vi "TMP007 Read.vi"(7 "I2C Channel":u8, 8 "error in (no error)":errorcluster, 10 "I2C Slave Address":u8 format="%.0x", 11 "LINX Resource in":T2) -> (0 "error out":errorcluster, 1 "Conversion Time (S)":dbl format="%#_g s", 2 "Temp Readings":T1 {"Ambient Temp (°F)" format="%.2f °F"; "Ambient Temp (°C)" format="%.2f °C"; "Object Temp (°F)" format="%.2f °F"; "Object Temp (°C)" format="%.2f °C"}, 3 "LINX Resource":T2)   [LabVIEW 2014]
uses:
  <vilib>/MakerHub/LINX/Private/Type Defs/LINX Ref.ctl
  <vilib>/MakerHub/LINX/Private/Type Defs/Platform.ctl
  <vilib>/MakerHub/LINX/Private/Type Defs/Interface.ctl
  <vilib>/MakerHub/LINX/Private/Device/Type Defs/LINX Device Config.ctl
  <vilib>/MakerHub/LINX/Private/Device/Type Defs/TCP Config.ctl
  <vilib>/MakerHub/LINX/Private/Device/Type Defs/Channels.ctl
  <vilib>/MakerHub/LINX/Private/Local IO/LinxI2cWrite.vi
  <vilib>/MakerHub/LINX/Public/Utilities/Check Channel.vi
  <vilib>/myRIO/Instrument Drivers/Onboard IO/I2C/vis/Write.vi
  <vilib>/MakerHub/LINX/Private/Utilties/Generate Error.vi
  <vilib>/MakerHub/LINX/Private/Utilties/Channel FGVs/I2C Channels.vi
  <vilib>/Utility/error.llb/Error Cluster From Error Code.vi
  <vilib>/myRIO/Common/Instrument Driver Framework/myRIO v1.0/I2C/vis/myRIO v1.0 Write I2C.vi
  <vilib>/MakerHub/LINX/LMH-LINX.lvlib
  <vilib>/MakerHub/LINX/Private/Device/Device.lvlib
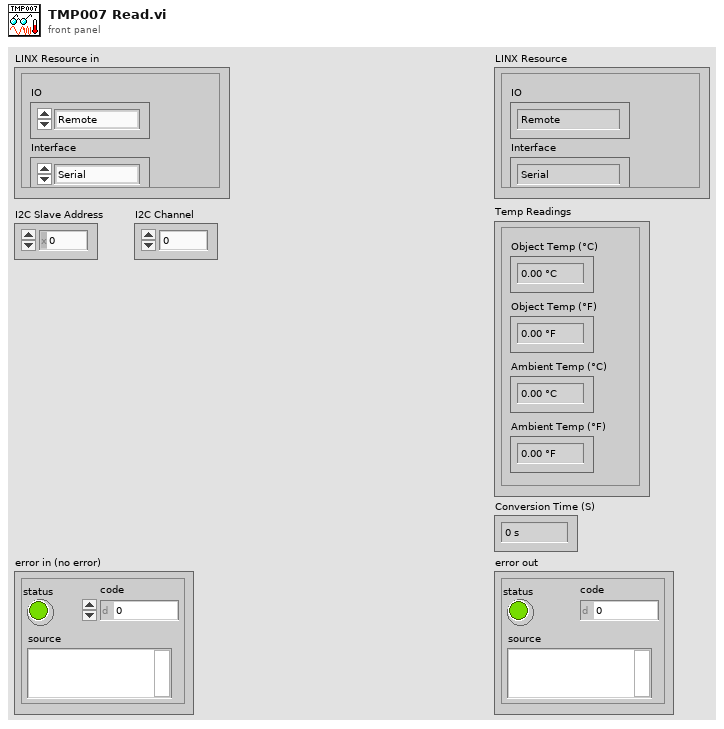
[diagram p1: front panel]
types:
  T1 = cluster{"Object Temp (°C)":dbl, "Object Temp (°F)":dbl, "Ambient Temp (°C)":dbl, "Ambient Temp (°F)":dbl}
  T2 = typedef "LMH-LINX.lvlib/LINX Ref.ctl" = cluster{"IO":T3, "Interface":T4, "LINX Device Config":T5}
  T3 = typedef "LMH-LINX.lvlib/Platform.ctl" = enum16{"Remote", "Local"}
  T4 = typedef "LMH-LINX.lvlib/Interface.ctl" = enum16{"Serial", "TCP"}
  T5 = typedef "LMH-LINX.lvlib/Device.lvlib/LINX Device Config.ctl" = cluster{"Interface":T4, "COM Port":refnum<visa-resource-name>, "TCP Configuration":T6, "Device Family":u8, "Device ID":u8, "Device Name":string, "TCP Ref":refnum<k5>, "Channels":T7}
  T6 = typedef "LMH-LINX.lvlib/Device.lvlib/TCP Config.ctl" = cluster{"IP Address":string, "Port":u16}
  T7 = typedef "LMH-LINX.lvlib/Channels.ctl" = cluster{"DI":u8[], "DO":u8[], "AI":u8[], "AO":u8[], "PWM":u8[], "QE":u8[], "UART":u8[], "I2C 2":u8[], "SPI":u8[], "CAN":u8[], "Servo":u8[], "AI Ref (V)":dbl, "AI Resolution (Bits)":u8, "AO Ref (V)":dbl, "AO Resolution (Bits)":u8}
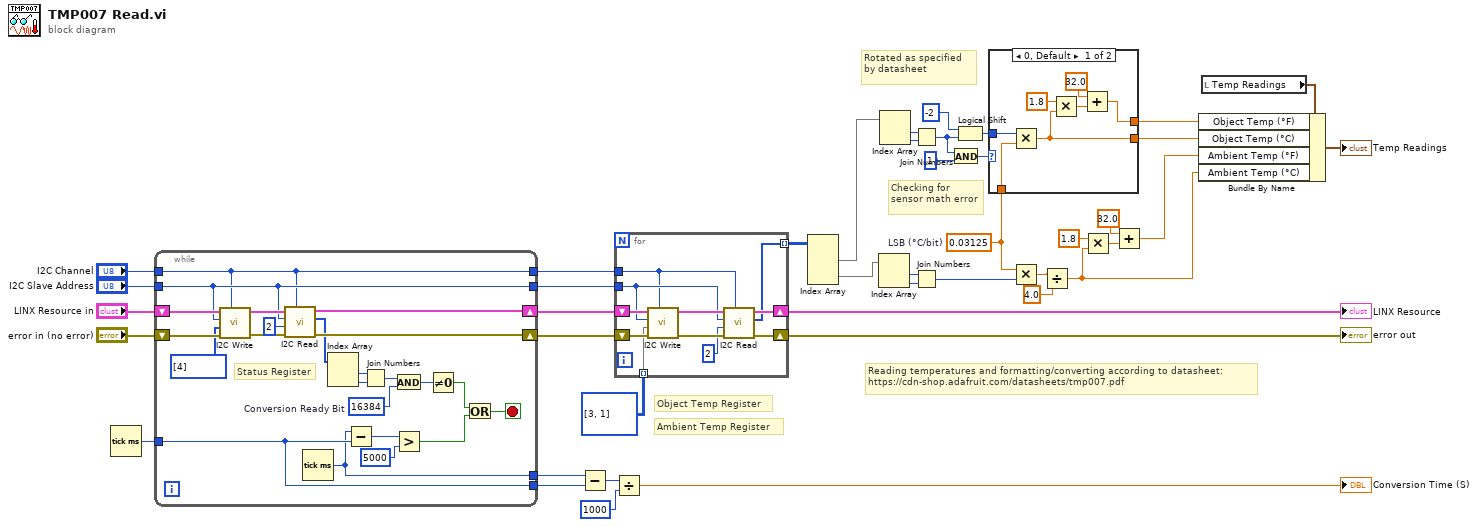
[diagram p0: block diagram]
diagram:
  w26 = 0.03125  # LSB (°C/bit)
  # "Reading temperatures and formatting/converting according to datasheet:\nhttps://cdn-shop.adafruit.com/datasheets/tmp007.pdf"
  # "Rotated as specified by datasheet"
  # "Checking for sensor math error"
  # "Ambient Temp Register"
  # "Object Temp Register"
  n1 = Tick Count (ms)() -> (millisecond timer value=w9:u32)
  n2 = while {
    tunnel: "I2C Channel" -> [w57]
    tunnel: "I2C Slave Address" -> [w58]
    tunnel: [w57] -> w11
    tunnel: [w58] -> w10
    shift-right: [w59] -> w15
    shift-left: "error in (no error)" -> [w64]
    shift-right: [w60] -> w14
    shift-left: "LINX Resource in" -> [w65]
    tunnel: w9 -> [w44]
    tunnel: [w44] -> w8
    tunnel: [w43] -> w4
    stop <- w46 stop-if-true
    w51 = u16 16384  # Conversion Ready Bit
    # "Status Register"
    n3 = call <vilib>:"I2C Write.vi"("I2C Channel"=w57, "Error In"=w64, "Data"=u8[] [4], "I2C Slave Address (0)"=w58, "LINX Resource"=w65) -> ("Error Out"=w61:errorcluster, "LINX Resource"=w62:T2)  [unwired: 5 in]
    n4 = call <vilib>:"I2C Read.vi"("I2C Channel"=w57, "Error In"=w61, "Bytes To Read"=u8 2, "I2C Slave Address (0)"=w58, "LINX Resource"=w62) -> ("Error Out"=w59:errorcluster, "Data"=w54:u8[], "LINX Resource"=w60:T2)  [unwired: 4 in]
    n5 = Tick Count (ms)() -> (millisecond timer value=w43:u32)
    n6 = Index Array(array=w54) -> (element #1=w55:u8, element #2=w53:u8)  [unwired: 2 in]
    n7 = Subtract(x=w43, y=w44) -> (x-y=w50:u32)
    n8 = Join Numbers(hi=w55, lo=w53) -> ((hi.lo)=w52:u16)
    n9 = And(x=w52, y=w51) -> (x .and. y?=w48:u16)
    n10 = Greater?(x=w50, y=u32 5000) -> (0:w47:bool)
    n11 = Not Equal To 0?(x=w48) -> (x != 0?=w45:bool)
    n12 = Or(x=w45, y=w47) -> (x .or. y?=w46:bool)
  }
  n13 = Subtract(x=w4, y=w8) -> (x-y=w7:u32)
  n14 = Divide(x=w7, y=u32 1000) -> (x/y=→"Conversion Time (S)":dbl)
  n15 = for {
    tunnel: w10 -> [w70]
    tunnel: w11 -> [w69]
    shift-right: [w71] -> w41
    shift-left: w15 -> [w76]
    shift-right: [w72] -> w42
    shift-left: w14 -> [w75]
    tunnel: u8[][] [[3], [1]] ("Data") -> [w67] mode=indexing
    tunnel: [w66] -> w39 mode=indexing
    n16 = call <vilib>:"I2C Write.vi"("I2C Channel"=w69, "Error In"=w76, "Data"=w67, "I2C Slave Address (0)"=w70, "LINX Resource"=w75) -> ("Error Out"=w73:errorcluster, "LINX Resource"=w74:T2)  [unwired: 5 in]
    n17 = call <vilib>:"I2C Read.vi"("I2C Channel"=w69, "Error In"=w73, "Bytes To Read"=u8 2, "I2C Slave Address (0)"=w70, "LINX Resource"=w74) -> ("Error Out"=w71:errorcluster, "Data"=w66:u8[], "LINX Resource"=w72:T2)  [unwired: 4 in]
  }
  "error out" <- w41
  "LINX Resource" <- w42
  n18 = Index Array(array=w39) -> (element #1=w38:u8[], element #2=w37:u8[])  [unwired: 4 in]
  n19 = Index Array(array=w37) -> (element #1=w34:u8, element #2=w33:u8)  [unwired: 2 in]
  n20 = Index Array(array=w38) -> (element #1=w35:u8, element #2=w36:u8)  [unwired: 2 in]
  n21 = Join Numbers(hi=w35, lo=w36) -> ((hi.lo)=w31:u16)
  n22 = Join Numbers(hi=w34, lo=w33) -> ((hi.lo)=w29:u16)
  n23 = And(x=w31, y=u16 1) -> (x .and. y?=w25:u16)
  n24 = Logical Shift(y=i16 -2, x=w31) -> (x << y=w27:u16)
  n25 = case shown="0, Default" w25 {
    tunnel: w27 -> [w83 _]
    tunnel: w26 -> [w82 _]
    tunnel: [w78 _] -> w24
    tunnel: [w77 _] -> w23
    frame 0, Default {
      n26 = Multiply(x=w83, y=w82) -> (x*y=w78:dbl)
      n27 = Multiply(x=1.8, y=w78) -> (x*y=w79:dbl)
      n28 = Add(x=32.0, y=w79) -> (x+y=w77:dbl)
    }
    frame 1 {
      # "Sensor math error found on sensor"
    }
  }
  n29 = Multiply(x=w26, y=w29) -> (x*y=w3:dbl)
  n30 = Divide(x=w3, y=4.0) -> (x/y=w2:dbl)
  n31 = Multiply(x=1.8, y=w2) -> (x*y=w22:dbl)
  n32 = Add(x=32.0, y=w22) -> (x+y=w19:dbl)
  n33 = local read "Temp Readings"() -> (w28:T1)
  n34 = Bundle By Name(cluster=w28, "Object Temp (°F)"=w23, "Object Temp (°C)"=w24, "Ambient Temp (°F)"=w19, "Ambient Temp (°C)"=w2) -> (→"Temp Readings":T1)
